vi "Choreo_TrajectorySwerve_SampleAt.vi"(9 "MirrorForRedAlliance":bool, 10 "TimeStamp":dbl, 11 "ChoreoTrajectorySwerve":T2) -> (3 "ChoreoSwerveSample":T1)   [LabVIEW 2019, in "ChoreoLib.lvlib"]
doc: "Return an interpolated sample of the trajectory at the given timestamp.\n\nInputs: \n - ChoreoTrajectory - cluster - The trajectory to sample.\n - timestamp - double - The timestamp of this sample relative to the beginning of the trajectory.\n - mirrorForRedAlliance - boolean - whether or not to return the sample as mirrored across the field midline (as in 2023). (Optional. Default: false )\n\nOutputs:\n - ChoreoTrajectoryState - cluster - The ChoreoTrajectoryState at the given time."
uses:
  ChoreoLib.lvlib
  TypeDef/ChoreoSwerveSample.ctl
  TypeDef/ChoreoEventMarker.ctl
  TypeDef/ChoreoTrajectorySwerve.ctl
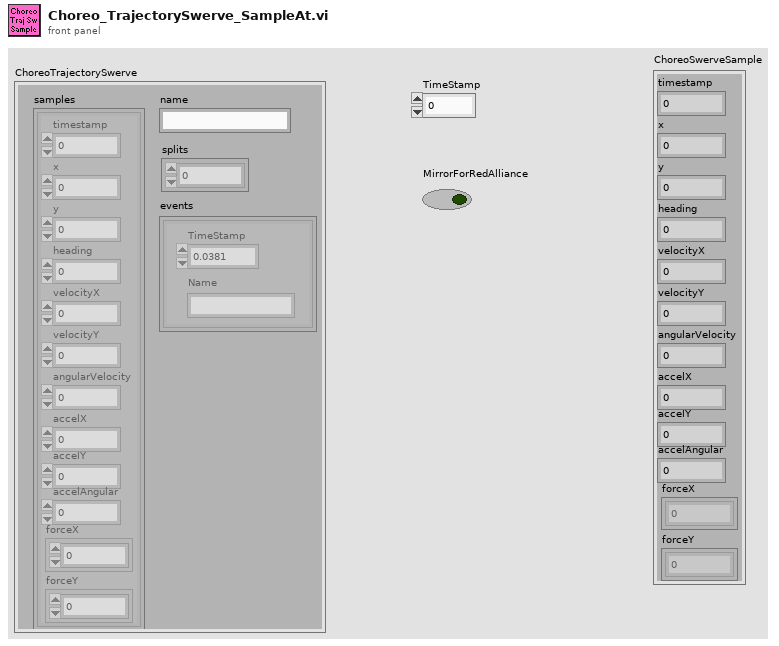
[diagram p1: front panel]
types:
  T1 = typedef "ChoreoLib.lvlib/ChoreoSwerveSample.ctl" = cluster{"timestamp":dbl, "x":dbl, "y":dbl, "heading":dbl, "velocityX":dbl, "velocityY":dbl, "angularVelocity":dbl, "accelX":dbl, "accelY":dbl, "accelAngular":dbl, "forceX":dbl[], "forceY":dbl[]}
  T2 = typedef "ChoreoLib.lvlib/ChoreoTrajectorySwerve.ctl" = cluster{"name":string, "samples":T1[], "splits":i32[], "events":T3[]}
  T3 = typedef "ChoreoLib.lvlib/ChoreoEventMarker.ctl" = cluster{"TimeStamp":dbl, "Name":string}
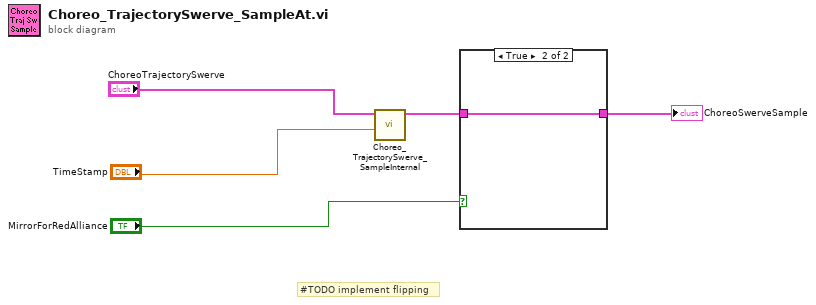
[diagram p0: block diagram]
diagram:
  # "#TODO implement flipping"
  n1 = call "Choreo_TrajectorySwerve_SampleInternal.vi"("TimeStamp"="TimeStamp", "ChoreoTrajectorySwerve"="ChoreoTrajectorySwerve") -> ("ChoreoSwerveSample"=w2:T1)  [unwired: 9 in]
  n2 = case shown="True" "MirrorForRedAlliance" {
    tunnel: w2 -> [w6 w7]
    tunnel: [w6 w7] -> w1
    frame False {
    }
    frame True {
    }
  }
  "ChoreoSwerveSample" <- w1
